vi "_Anritsu_SA_Write.vi"(6 "Comand":string="FREQ:CENT 5GHZ", 7 "address":string="192.168.0.6") -> (0 "error out":errorcluster)   [LabVIEW 2013]
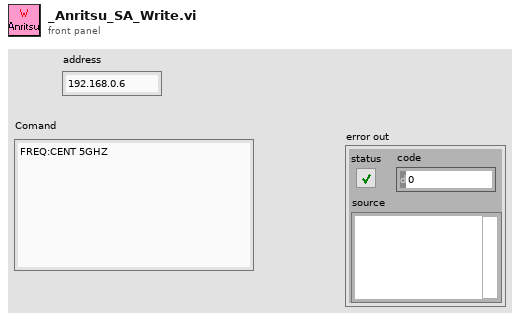
[diagram p1: front panel]
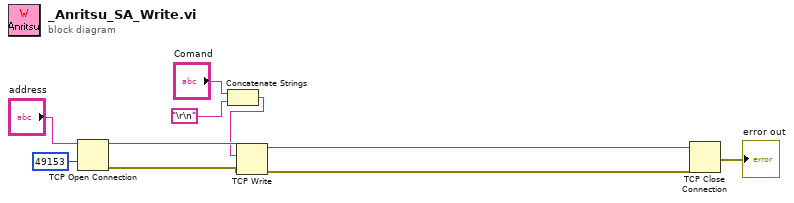
[diagram p0: block diagram]
diagram:
  n1 = TCP Open Connection(address="address", remote port or service name=u16 49153) -> (connection ID=w10:refnum<k5>, error out=w9:errorcluster)  [unwired: 3 in]
  n2 = Concatenate Strings("Comand", "\r\n") -> (w3:string)
  n3 = TCP Write(connection ID=w10, data in=w3, error in (no error)=w9) -> (connection ID out=w2:refnum<k5>, error out=w1:errorcluster)  [unwired: 1 in, 1 out]
  n4 = TCP Close Connection(connection ID=w2, error in (no error)=w1) -> (error out=→"error out":errorcluster)  [unwired: 1 in, 1 out]
